vi "GenerateListOfCoordintes (SubVI).vi"(0 "Module side length [mm]":dbl=97.54, 1 "Nloops":i32=1, 2 "A [mm]":cluster{"X":dbl, "Y":dbl, "Z":dbl}={"X"=122.518, "Y"=-50.0451, "Z"=10.3689}, 3 "x to fiducial [um]":dbl=980.0, 4 "y to fiducial [um]":dbl=980.0) -> (7 "Generated List of Coordinates":dbl[][](array[numeric])=[[122.518, -50.0451, 10.3689], [218.098, -50.0451, 10.3689], [218.098, -145.6251, 10.3689], [122.518, -145.6251, 10.3689]])   [LabVIEW 2016]
uses:
  <vilib>/Utility/file.llb/Write Delimited Spreadsheet (DBL).vi
panel:
  in  "file path (dialog if empty)":path=path "C:/Users/Aerotech/Documents/Stave Assembly Records/2017-03-30/ChangeHeight/corners.csv"
  out "D [mm]":cluster{"X":dbl, "Y":dbl, "Z":dbl}={"X"=122.518, "Y"=-145.6251, "Z"=10.3689}
  out "C [mm]":cluster{"X":dbl, "Y":dbl, "Z":dbl}={"X"=218.098, "Y"=-145.6251, "Z"=10.3689}
  out "B [mm]":cluster{"X":dbl, "Y":dbl, "Z":dbl}={"X"=218.098, "Y"=-50.0451, "Z"=10.3689}
  out "lv [mm]":dbl=95.58
  out "lh [mm]":dbl=95.58
  # "2*230 um for 4dots"
  # "2*(230+300+500) um for 4dots"
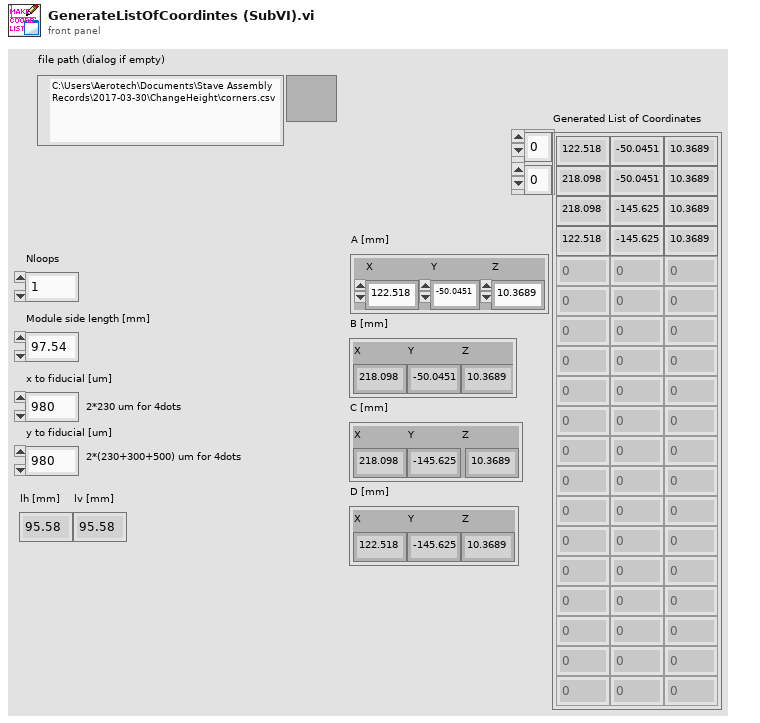
[diagram p1: front panel]
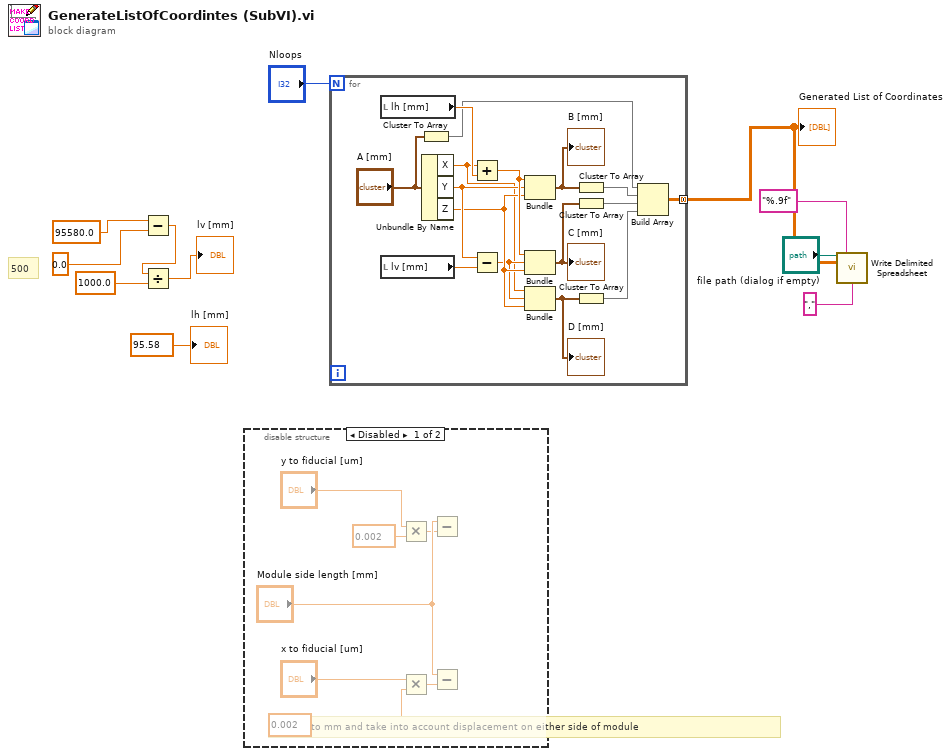
[diagram p0: block diagram]
diagram:
  # "500"
  # "Convert to mm and take into account displacement on either side of module"
  n1 = Subtract(x=95580.0 ("lv [mm]"), y=0.0) -> (x-y=w2:dbl)
  n2 = Divide(x=w2, y=1000.0) -> (x/y=→"lv [mm]":dbl)
  n3 = disable-structure shown="Disabled" {
    frame Disabled {
      n4 = Multiply(x="y to fiducial [um]", y=0.002) -> (x*y=w13:dbl)
      n5 = Multiply(x="x to fiducial [um]", y=0.002) -> (x*y=w16:dbl)
      n6 = Subtract(x="Module side length [mm]", y=w13) -> (x-y=w12:dbl)
      n7 = Subtract(x="Module side length [mm]", y=w16) -> (x-y=w15:dbl)
    }
    frame Enabled {
    }
  }
  n8 = for {
    N: "Nloops" -> [_]
    tunnel: [w21] -> w10 mode=concatenating
    n9 = local read "lh [mm]"() -> (w36:dbl)
    n10 = local read "lv [mm]"() -> (w33:dbl)
    n11 = Cluster To Array(cluster="A [mm]") -> (array=w28:dbl[])
    n12 = Unbundle By Name("A [mm]") -> ("X"=w30:dbl, "Y"=w34:dbl, "Z"=w32:dbl)
    n13 = Add(x=w30, y=w36) -> (x+y=w35:dbl)
    n14 = Subtract(x=w34, y=w33) -> (x-y=w31:dbl)
    n15 = Bundle(w35, "Y"=w34, "Z"=w32) -> (w27:cluster{dbl, "Y":dbl, "Z":dbl})  [unwired: 1 in]
    "B [mm]" <- w27
    n16 = Bundle(w35, w31, "Z"=w32) -> (w26:cluster{dbl, dbl, "Z":dbl})  [unwired: 1 in]
    "C [mm]" <- w26
    n17 = Bundle("X"=w30, w31, "Z"=w32) -> (w25:cluster{"X":dbl, dbl, "Z":dbl})  [unwired: 1 in]
    "D [mm]" <- w25
    n18 = Cluster To Array(cluster=w27) -> (array=w24:dbl[])
    n19 = Cluster To Array(cluster=w26) -> (array=w23:dbl[])
    n20 = Cluster To Array(cluster=w25) -> (array=w22:dbl[])
    n21 = Build Array(w28, w24, w23, w22) -> (w21:dbl[][])
  }
  "Generated List of Coordinates" <- w10
  n22 = call-poly <vilib>:"Write Delimited Spreadsheet.vi"("file path (dialog if empty)"="file path (dialog if empty)", "format (%.3f)"="%.9f", "2D data"=w10, "delimiter (\\t)"="," ("delimiter (\\t)")) -> ()  [unwired: 10 in, 2 out]
  "lh [mm]" <- 95.58 ("lh [mm]")
